vi "simulatorCustomFeedbackControl.vi"(8 "error in (no error)":errorcluster, 10 "RobotsFeedback":refnum<class "RobotFeedback.lvclass">[](array[class]), 11 "Communication in":refnum<class "Communication.lvclass">) -> (0 "error out":errorcluster, 2 "feedback_array":refnum<class "RobotFeedback.lvclass">[](array[class]), 3 "Communication out":refnum<class "Communication.lvclass">)   [LabVIEW 2021, in "Communication.lvclass"]
uses:
  Communication.lvclass
  RobotFeedback/RobotFeedback.lvclass
  RobotFeedback/RobotFeedback.lvclass/RobotFeedback.ctl
  <vilib>/Analysis/_algsub.llb/Real PseudoInverse Matrix.vi
  <vilib>/Analysis/baseanly.llb/A x Vector.vi
  RobotFeedback/Write id.vi
  <vilib>/Analysis/NI_AALBase.lvlib
  <vilib>/Analysis/NI_AALPro.lvlib
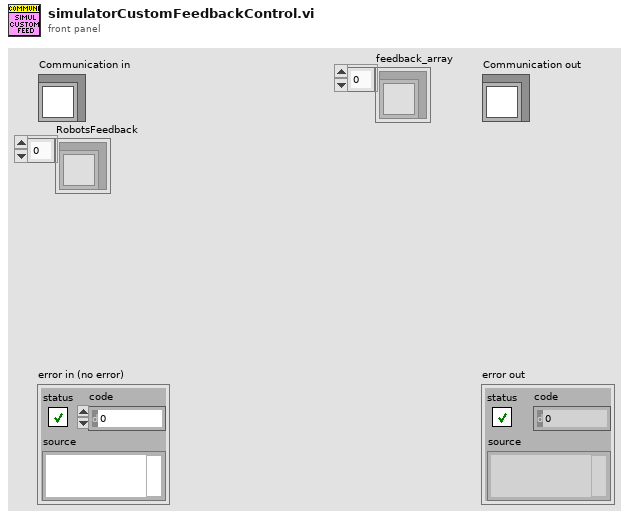
[diagram p1: front panel]
types:
  T1 = typedef "NI_Matrix.lvlib/RealMatrix.ctl" = dbl[][]
  T2 = typedef "feedbackData.ctl" = cluster{"id":u32, "status":u32, "battery":sgl, "encoder1":sgl, "encoder2":sgl, "encoder3":sgl, "encoder4":sgl}
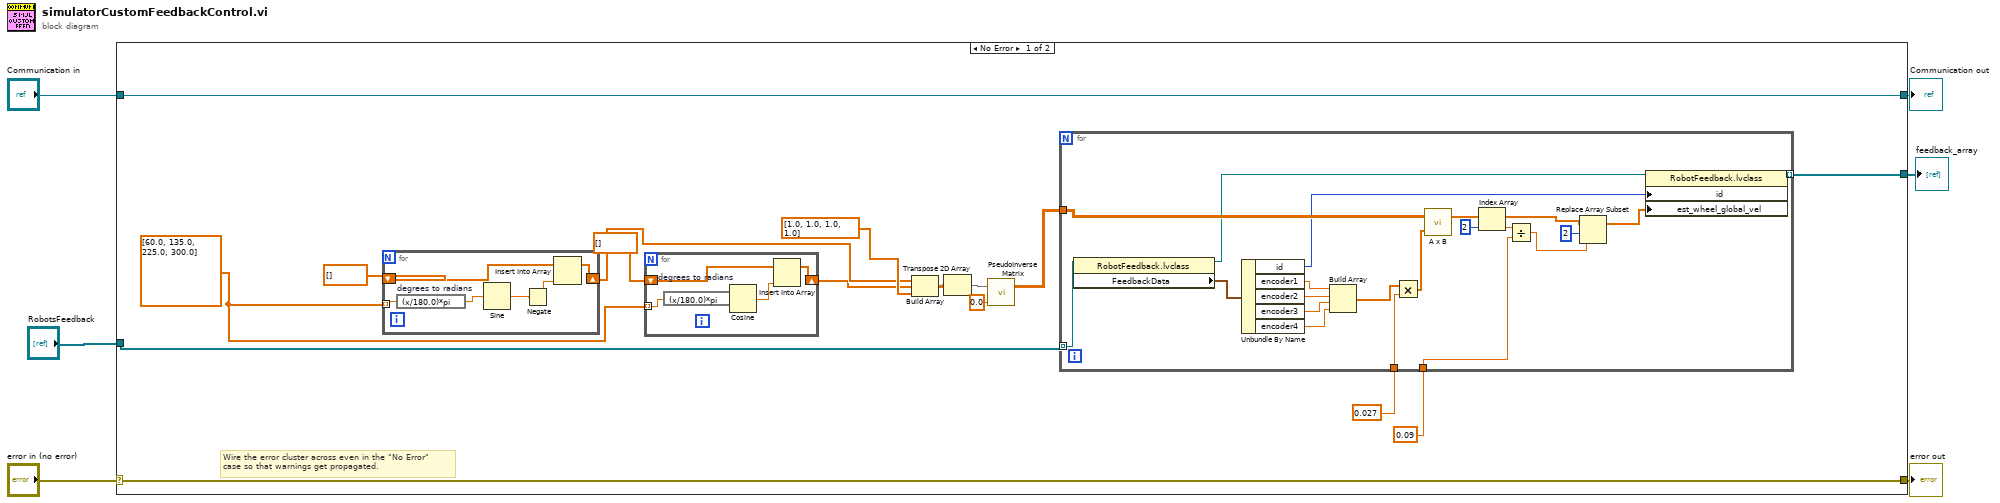
[diagram p0: block diagram]
diagram:
  n1 = case shown="No Error" "error in (no error)" {
    selector: "error in (no error)" -> [w21 w55]
    tunnel: [w21 w55] -> w5
    tunnel: [w22 w54] -> w3
    tunnel: "Communication in" -> [w22 w54]
    tunnel: "RobotsFeedback" -> [w10 _]
    tunnel: [w7 _] -> w1
    frame No Error {
      w20 = dbl[] [60.0, 135.0, 225.0, 300.0] ("robotAngles 2")
      # "Wire the error cluster across even in the \"No Error\"\ncase so that warnings get propagated."
      n2 = for {
        shift-right: [w52] -> w12
        shift-left: dbl[] [] -> [w53]
        tunnel: w20 -> [w51] mode=indexing
        n3 = expression code="(x/180.0)*pi" "degrees to radians"(w51) -> (w50:dbl)
        n4 = Sine(x=w50) -> (sin(x)=w49:dbl)
        n5 = Negate(x=w49) -> (-x=w48:dbl)
        n6 = Insert Into Array(array=w53, new element=w48) -> (w52:dbl[])  [unwired: 1 in]
      }
      n7 = for {
        shift-right: [w46] -> w11
        shift-left: dbl[] [] -> [w47]
        tunnel: w20 -> [w45] mode=indexing
        n8 = expression code="(x/180.0)*pi" "degrees to radians"(w45) -> (w44:dbl)
        n9 = Cosine(x=w44) -> (cos(x)=w43:dbl)
        n10 = Insert Into Array(array=w47, new element=w43) -> (w46:dbl[])  [unwired: 1 in]
      }
      n11 = Build Array(w12, w11, dbl[] [1.0, 1.0, 1.0, 1.0] ("Numeric")) -> (w16:dbl[][])
      n12 = Transpose 2D Array(2D array=w16) -> (transposed array=w15:dbl[][])
      n13 = call-poly <vilib>:"PseudoInverse Matrix.vi"("tolerance"=0.0, "Input Matrix"=w15) -> ("PseudoInverse Matrix"=w14:T1)  [unwired: 1 out]
      n14 = for {
        tunnel: w10 -> [w42] mode=indexing
        tunnel: w14 -> [w41]
        tunnel: 0.027 ("r_wheel") -> [w40]
        tunnel: 0.09 ("r_robot") -> [w34]
        tunnel: [w23] -> w7 mode=indexing
        n15 = property class="RobotFeedback.lvclass"(reference=w42) -> (reference out=w26:refnum<class "RobotFeedback.lvclass">, "FeedbackData"=w27:T2)  [unwired: 1 in, 1 out]
        n16 = Unbundle By Name(w27) -> ("id"=w24:u32, "encoder1"=w32:sgl, "encoder2"=w31:sgl, "encoder3"=w30:sgl, "encoder4"=w29:sgl)
        n17 = Build Array(w32, w31, w30, w29) -> (w28:sgl[])
        n18 = Multiply(x=w28, y=w40) -> (x*y=w39:dbl[])
        n19 = call-poly <vilib>:"A x B.vi"("Vector"=w39, "A"=w41) -> ("A x Vector"=w37:dbl[])  [unwired: 1 out]
        n20 = Index Array(array=w37, index=2) -> (element=w35:dbl)
        n21 = Divide(x=w35, y=w34) -> (x/y=w33:dbl)
        n22 = Replace Array Subset(array=w37, new element=w33, index=2) -> (w25:dbl[])
        n23 = property class="RobotFeedback.lvclass"(reference=w26, "id"=w24, "est_wheel_global_vel"=w25) -> (reference out=w23:refnum<class "RobotFeedback.lvclass">)  [unwired: 1 in, 1 out]
      }
    }
    frame Error {
    }
  }
  "error out" <- w5
  "Communication out" <- w3
  "feedback_array" <- w1
